vi "LoadFpgaWithData.vi"(7 "subband_sample_rate":dbl, 8 "ChirpFftPairs":T1(array[cluster]), 9 "num_cfft":i32, 10 "DataIn":csg[](array[numeric]), 11 "NumDataPoints":i32) -> (3 "Return Value":i32)   [LabVIEW 2014]
uses:
  LV_FGV/SETI_LV_FGV.ctl
  SETI_LV/SETI_LV.lvlib
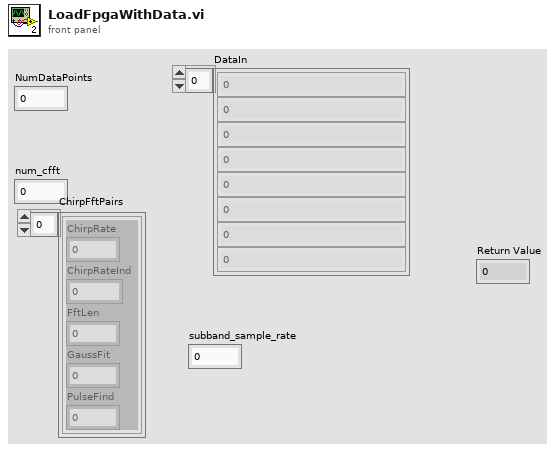
[diagram p1: front panel]
types:
  T1 = cluster{"ChirpRate":dbl, "ChirpRateInd":i32, "FftLen":i32, "GaussFit":i32, "PulseFind":i32}[]
  T2 = typedef "SETI_LV.lvlib/SETI_LV_FGV.ctl" = enum16{"Get", "Set", "Chirp(icfft)"}
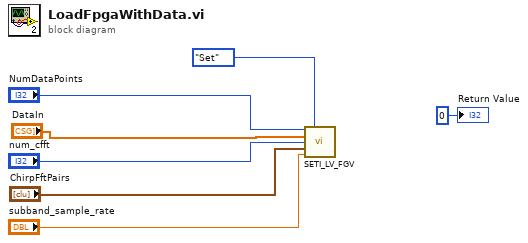
[diagram p0: block diagram]
diagram:
  n1 = call "SETI_LV_FGV.vi"("NumDataPoints in"="NumDataPoints", "Command"=SETI_LV_FGV."Set", "DataIn in"="DataIn", "num_cfft in"="num_cfft", "Chirp FFT Pairs in"="ChirpFftPairs", "subband_sample_rate in"="subband_sample_rate") -> ()  [unwired: 5 in, 5 out]
  "Return Value" <- 0 ("Return Value")
